vi "Report_SetTableColumnWidth.vi"(6 "MeasurementSystem":i32(ring) items=["Default", "US", "Metric"], 8 "error in":errorcluster, 9 "Column Width":dbl[](array[numeric]) format="%.2f", 11 "AppendTable":refnum<k7>) -> (0 "error out":errorcluster)   [LabVIEW 2020]
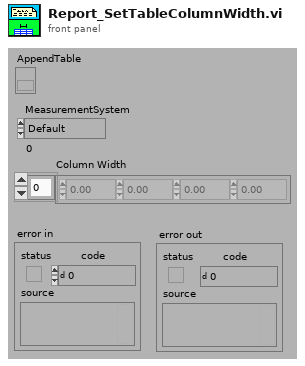
[diagram p1: front panel]
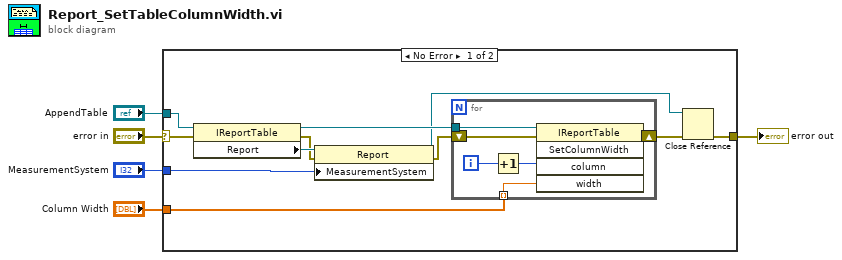
[diagram p0: block diagram]
diagram:
  n1 = case shown="No Error" "error in" {
    selector: "error in" -> [w6 w23]
    tunnel: "AppendTable" -> [w12 _]
    tunnel: "MeasurementSystem" -> [w11 _]
    tunnel: [w10 w23] -> w3
    tunnel: "Column Width" -> [w7 _]
    frame No Error {
      n2 = property class="IReportTable"(reference=w12, error in=w6) -> (reference out=w13:refnum<k7>, error out=w14:errorcluster, "Report"=w16:refnum<k7>)
      n3 = property class="Report"(reference=w16, error in=w14, "MeasurementSystem"=w11) -> (reference out=w8:refnum<k7>, error out=w15:errorcluster)
      n4 = for {
        tunnel: w13 -> [w22]
        shift-right: [w19] -> w9
        shift-left: w15 -> [w18]
        tunnel: w7 -> [w17] mode=indexing
        i -> [w21]
        n5 = Increment(x=w21) -> (x+1=w20:i32)
        n6 = invoke class="IReportTable" method="SetColumnWidth"(reference=w22, error in=w18, "column"=w20, "width"=w17) -> (error out=w19:errorcluster)  [unwired: 1 in, 4 out]
      }
      n7 = Close Reference(reference=w8, error in (no error)=w9) -> (error out=w10:errorcluster)
    }
    frame Error {
    }
  }
  "error out" <- w3
